vi "Actor Core.vi"(8 "error in":errorcluster, 11 "State in":refnum<class "Command State Actor.lvclass">) -> (0 "error out":errorcluster, 3 "Actor out":refnum<class "Actor.lvclass">)   [LabVIEW 2013, in "Command State Actor.lvlib" / "Command State Actor.lvclass"]
doc: "(<B>Filename</B>: Actor Framework.lvlib:Actor.lvclass:Actor Core.vi)\n\nThis override invokes Entry.vi on the initial state, prior to calling the parent Actor Core. Adding this behavior to Actor Core (instead of an override of Pre Launch Init.vi) allows the initial state to launch a nested actor as part of its entry behavior.\n\nReceives messages to the actor, reacts to them, and initiates any error handling that may shut the actor down.\n\nDescendant classes may override this VI to append parallel tasks for the actor to complete while it handles messages. Overrides use the Call Parent Method node."
uses:
  Command State Actor.lvclass
  <vilib>/ActorFramework/Actor/Actor.lvclass
  Command Status.ctl
  Command States.ctl
  State Status.ctl
  Command State Actor.lvclass/Command State Actor.ctl
  <vilib>/ni/Actors/State Actor/State Actor/State Actor.lvclass
  Command Actor/Command States/Command States.lvclass
panel:
  in  "Command Status":T1
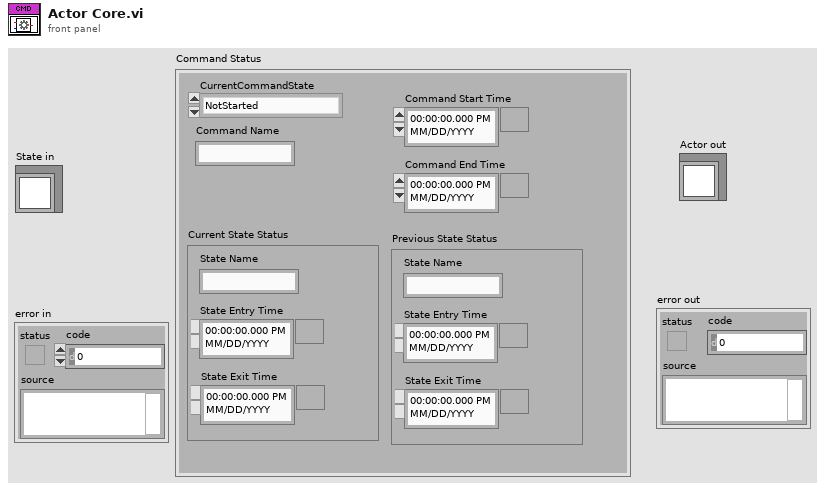
[diagram p1: front panel]
types:
  T1 = typedef "Command State Actor.lvlib/Command State Actor.lvclass/Command Status.ctl" = cluster{"CurrentCommandState":T2, "Command Name":string, "Current State Status":T3, "Command Start Time":timestamp, "Command End Time":timestamp, "Previous State Status":T3}
  T2 = typedef "Command State Actor.lvlib/Command State Actor.lvclass/Command States.ctl" = enum16{"NotStarted", "Starting", "Started", "Executing", "Completing", "Completed", "Stopping", "Stopped"}
  T3 = typedef "Command Actor.lvlib/Command States.lvclass/State Status.ctl" = cluster{"State Name":string, "State Entry Time":timestamp, "State Exit Time":timestamp}
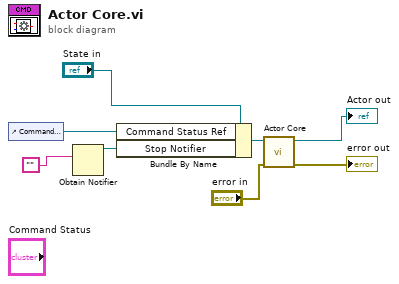
[diagram p0: block diagram]
diagram:
  n1 = control-ref of="Command Status"() -> (w3:refnum<vi>)
  n2 = Obtain Notifier(notification data type="") -> (notifier out=w2:refnum<notifier>)  [unwired: 3 in, 2 out]
  n3 = Bundle By Name(cluster="State in", "Command Status Ref"=w3, "Stop Notifier"=w2) -> (w4:refnum<class "Command State Actor.lvclass">)
  n4 = call-parent "Actor Core.vi"("error in"="error in", "State in"=w4) -> ("error out"=→"error out":errorcluster, "Actor out"=→"Actor out":refnum<class "Actor.lvclass">)  [unwired: 8 in]
